vi "Queue Reference.vi"(7 "Mode":T1(ring), 8 "Error In":errorcluster, 10 "Queue In":refnum<queue>, 11 "Name":string) -> (0 "Error Out":errorcluster caption="错误输出", 1 "Found?":bool, 2 "Queue Out":refnum<queue>, 3 "All Queue":map{string, refnum<queue>}(c390))   [LabVIEW 2020]
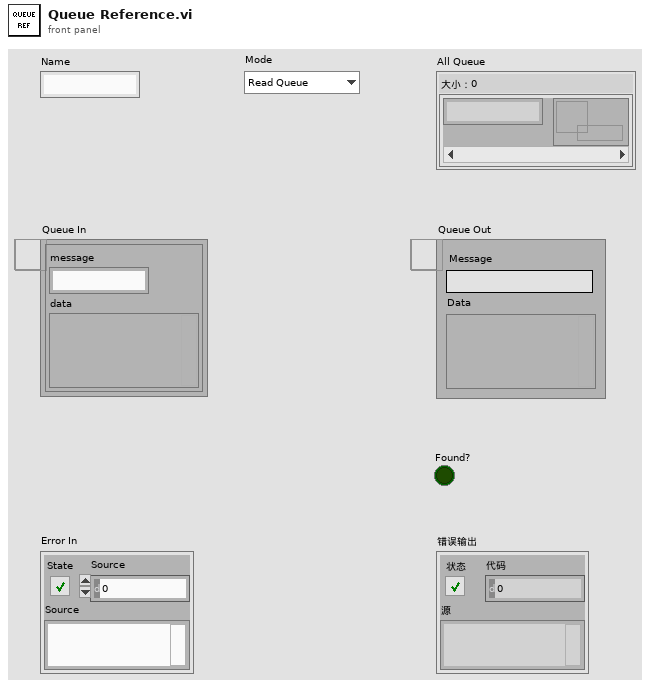
[diagram p1: front panel]
types:
  T1 = enum16{"Read Queue", "Add Queue", "Delete Queue"}
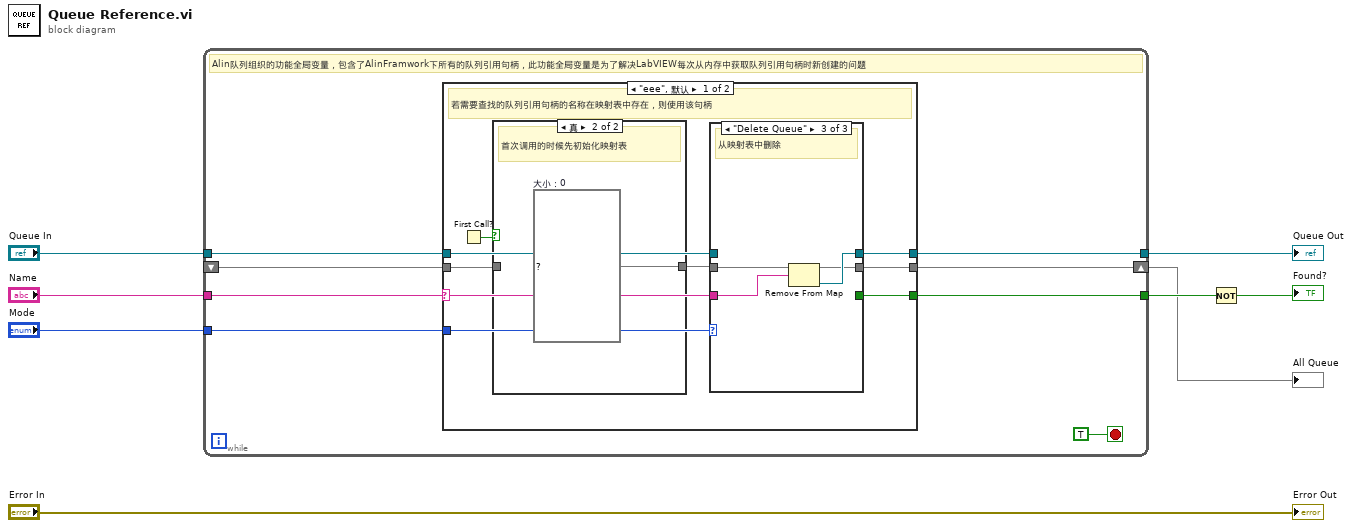
[diagram p0: block diagram]
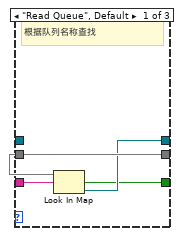
[diagram p2: hidden frame]
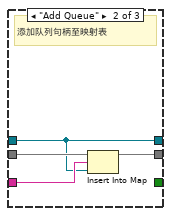
[diagram p3: hidden frame]
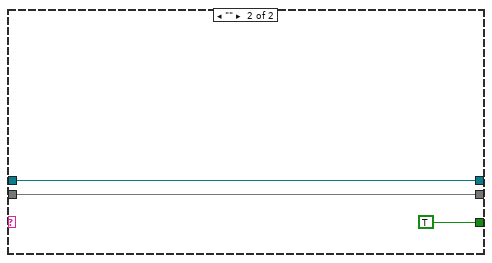
[diagram p5: hidden frame]
diagram:
  n1 = while {
    shift-right: [w9] -> w1
    shift-left: _ -> [w10]
    tunnel: "Name" -> [w15]
    tunnel: "Queue In" -> [w14]
    tunnel: "Mode" -> [w13]
    tunnel: [w12] -> w4
    tunnel: [w11] -> w3
    stop <- TRUE stop-if-true
    # "Alin队列组织的功能全局变量，包含了AlinFramwork下所有的队列引用句柄，此功能全局变量是为了解决LabVIEW每次从内存中获取队列引用句柄时新创建的问题"
    n2 = case shown="\"eee\", 默认" w15 {
      selector: w15 -> [w25 _]
      tunnel: w14 -> [w24 w42]
      tunnel: w13 -> [w23 _]
      tunnel: [w22 w42] -> w12
      tunnel: [w21 TRUE ("key not found?")] -> w11
      tunnel: w10 -> [w20 w41]
      tunnel: [w17 w41] -> w9
      frame "eee", Default {
        # "若需要查找的队列引用句柄的名称在映射表中存在，则使用该句柄"
        n3 = First Call?() -> (First Call?: T/F=w18:bool)
        n4 = case shown="真" w18 {
          tunnel: w20 -> [w38 _]
          tunnel: [w38 w39] -> w19
          frame False {
          }
          frame True {
            w39 = map{string, refnum<queue>} {}  # 大小：0
            # "首次调用的时候先初始化映射表"
          }
        }
        n5 = case shown="\"Delete Queue\"" w23 {
          tunnel: [w28 w33 w34] -> w17
          tunnel: w19 -> [w28 w32 w37]
          tunnel: w25 -> [w29 w31 w36]
          tunnel: w24 -> [_ w30 _]
          tunnel: [w27 w30 w35] -> w22
          tunnel: [w26 _ _] -> w21
          frame "Read Queue", Default {
            # "根据队列名称查找"
            n6 = Look In Map(map=w28, key=w29) -> (key not found?=w26:bool, value=w27:refnum<queue>)  [unwired: 1 in]
          }
          frame "Add Queue" {
            # "添加队列句柄至映射表"
            n7 = Insert Into Map(map in=w32, key=w31, value=w30) -> (map out=w33:map{string, refnum<queue>})  [unwired: 2 out]
          }
          frame "Delete Queue" {
            # "从映射表中删除"
            n8 = Remove From Map(10:w36, 11:w37) -> (1:w35:refnum<queue>, 3:w34:map{string, refnum<queue>})  [unwired: 1 out]
          }
        }
      }
      frame "" {
      }
    }
  }
  "Queue Out" <- w4
  "All Queue" <- w1
  n9 = Not(x=w3) -> (.not. x?=→"Found?":bool)
  "Error Out" <- "Error In"
